vi "Pcre2MakeTablesFree8.vi"(8 "error in":errorcluster, 11 "pTable":u64 format="%.0x") -> (0 "error out":errorcluster)   [LabVIEW 2021, in "libpcre2-8.lvlib"]
uses:
  libpcre2-8.lvlib
  libpcre2-8-x32.dll
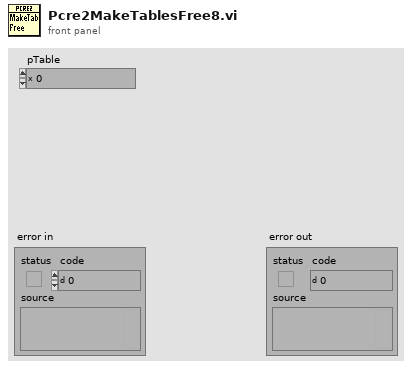
[diagram p1: front panel]
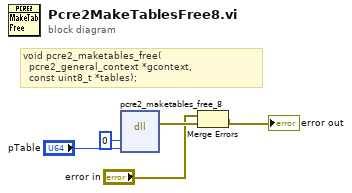
[diagram p0: block diagram]
diagram:
  # "void pcre2_maketables_free(\n  pcre2_general_context *gcontext,\n  const uint8_t *tables);"
  n1 = dll-call lib="libpcre2-8-x*.dll" fn="pcre2_maketables_free_8"("ctx"=u64 0, "pTable"="pTable") -> (error out=w3:errorcluster)  [unwired: 6 in, 1 out]
  n2 = Merge Errors("error in", w3) -> (→"error out":errorcluster)
